vi "HFCalibrate.vi"(7 "error in (no error)":errorcluster, 10 "VISA resource name":refnum<visa-resource-name>) -> (0 "error out":errorcluster, 1 "Calibrated freq / Hz":dbl, 2 "Calibration factor":dbl, 3 "VISA resource name out":refnum<visa-resource-name>)   [LabVIEW 2017, in "GP22_TDC_Arduinoed.lvlib"]
doc: "Calibrate the high frequency clokc by comparing it to the low freq but very stable 32.768 kHz clock.\n\nThis stores and returns a correction factor for the HF clock: e.g. if the clock is nominally 4MHz with a correction factor of 1.005, the true freq. is 4.02MHz. \n\nThe return value can be safely ignored: it is automatically stored and used by the measurement subVIs to calibrate their readings.\n\nCompared to the TDC calibration, this takes much longer and should be performed less often. TDC calibration should be carried out every few hundred measurements, but HF resonator calibration needs only to be done at the start of a measurement run. \n\nNote that this calibration is not handled automatically by the GP22 chip evenin \"autocalibrate\" mode, and so is dealt with by Labview."
uses:
  GP22_TDC_Arduinoed.lvlib
  Globals.vi
panel:
  out "read buffer":string
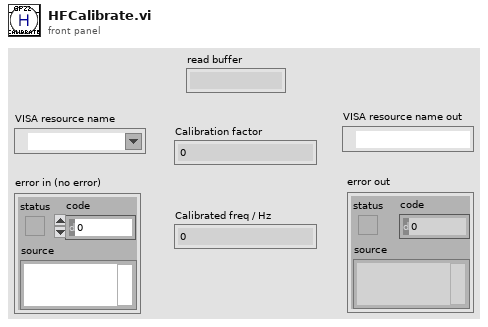
[diagram p1: front panel]
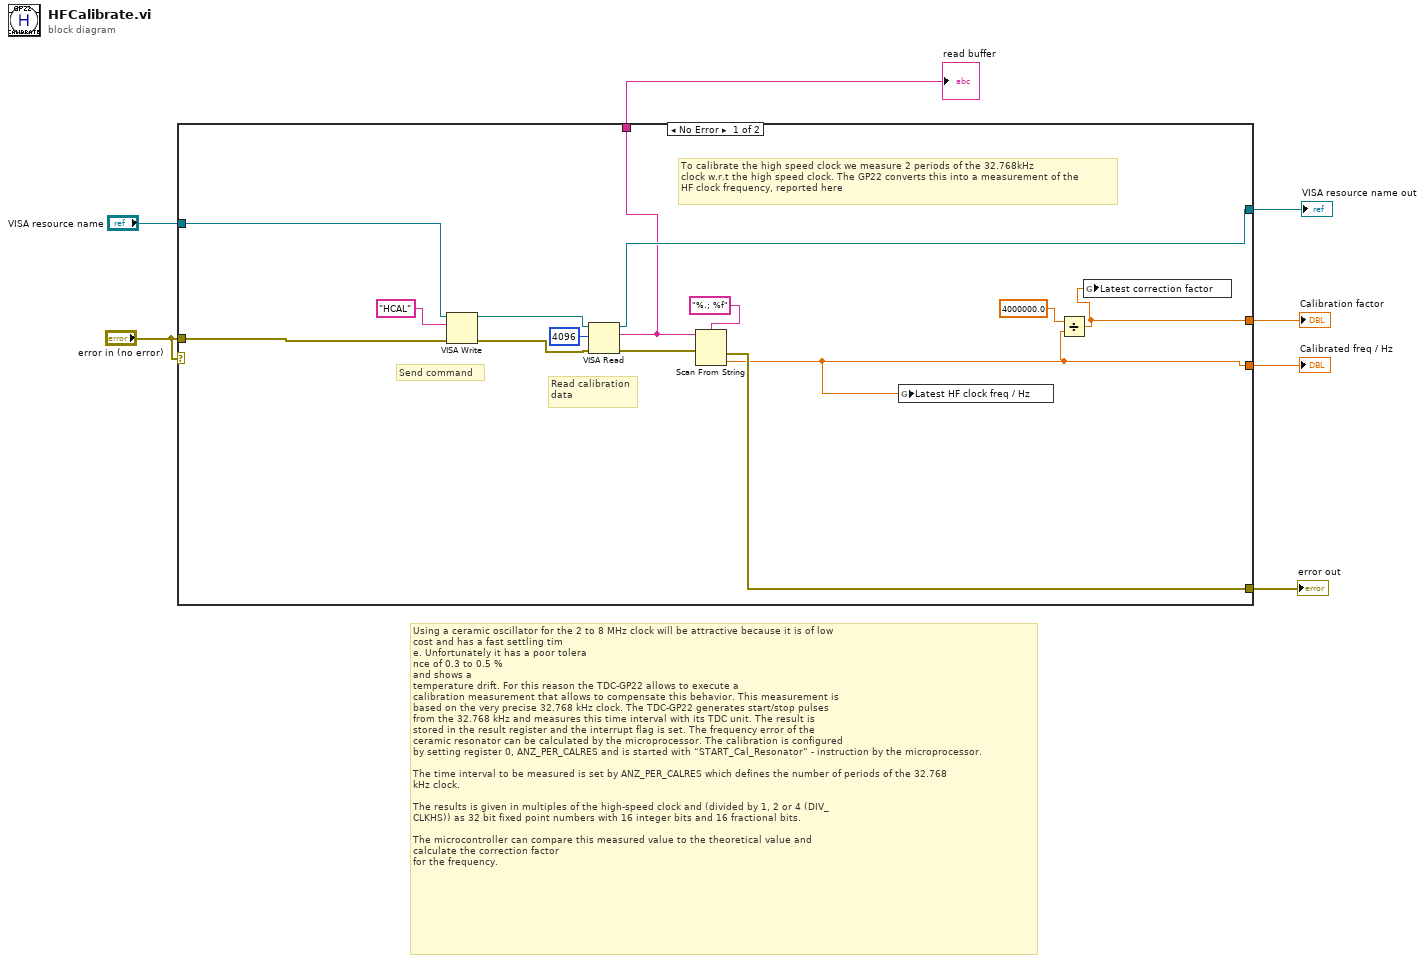
[diagram p0: block diagram]
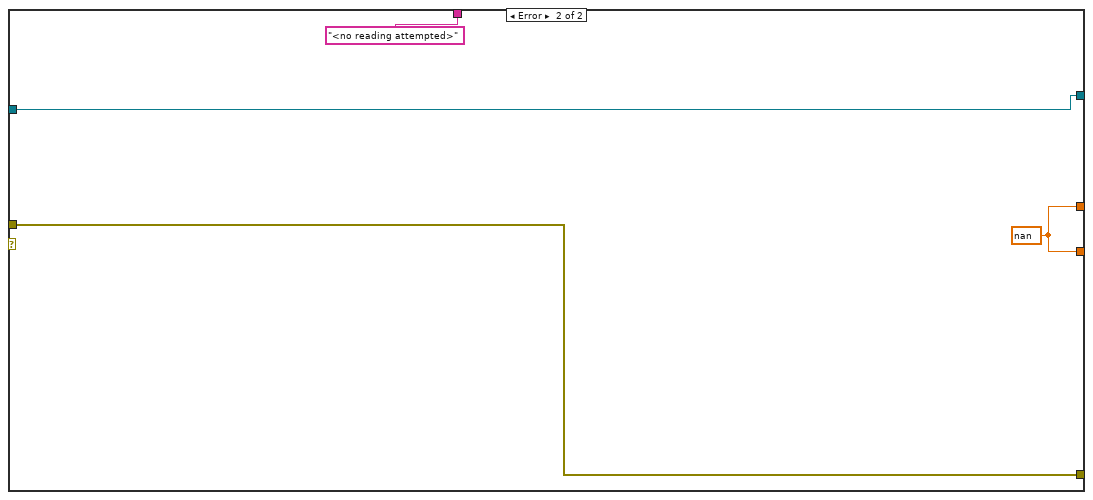
[diagram p2: hidden frame]
diagram:
  # "Using a ceramic oscillator for the 2 to 8 MHz clock will be attractive because it is of low\ncost and has a fast settling tim\ne. Unfortunately it has a poor tolera\nnce of 0.3 to 0.5 %\nand shows a\ntemperature drift. For this reason the TDC-GP22 allows to execute a\ncalibration measurement that allows to compensate this behavior. This measurement is\nbased on the very precise 32.768 kHz clock. The TDC-GP22 generates start/stop pulses\nfrom the 32.768 kHz and measures this time interval with its TDC unit. The result is\nstored in the result register and the interrupt flag is set. The frequency error of the\nceramic resonator can be calculated by the microprocessor. The calibration is configured\nby setting register 0, ANZ_PER_CALRES and is started with “START_Cal_Resonator“ - instruction by the microprocessor.\n\nThe time interval to be measured is set by ANZ_PER_CALRES which defines the number of periods of the 32.768\nkHz clock.\n\nThe results is given in multiples of the high-speed clock and (divided by 1, 2 or 4 (DIV_\nCLKHS)) as 32 bit fixed point numbers with 16 integer bits and 16 fractional bits.\n\nThe microcontroller can compare this measured value to the theoretical value and\ncalculate the correction factor\nfor the frequency."
  n1 = case shown="No Error" "error in (no error)" {
    tunnel: "error in (no error)" -> [w21 w25]
    tunnel: [w15 w25] -> w7
    tunnel: "VISA resource name" -> [w13 w23]
    tunnel: [w12 w23] -> w4
    tunnel: [w11 "<no reading attempted>" ("read buffer")] -> w3
    tunnel: [w8 w24] -> w2
    tunnel: [w9 w24] -> w1
    frame No Error {
      # "To calibrate the high speed clock we measure 2 periods of the 32.768kHz\nclock w.r.t the high speed clock. The GP22 converts this into a measurement of the\nHF clock frequency, reported here"
      # "Read calibration\ndata"
      # "Send command"
      n2 = VISA Write(VISA resource name=w13, write buffer="HCAL" ("command"), error in (no error)=w21) -> (VISA resource name out=w14:refnum<visa-resource-name>, error out=w20:errorcluster)  [unwired: 1 out]
      n3 = VISA Read(VISA resource name=w14, byte count=u32 4096, error in (no error)=w20) -> (VISA resource name out=w12:refnum<visa-resource-name>, read buffer=w11:string, error out=w16:errorcluster)  [unwired: 1 out]
      n4 = Scan From String(format string="%.; %f", input string=w11, error in=w16) -> (error out=w15:errorcluster, output 1=w9:dbl)  [unwired: 2 in, 2 out]
      n5 = global write "Globals.vi" "Latest HF clock freq / Hz"(w9) -> ()
      n6 = Divide(x=4000000.0, y=w9) -> (x/y=w8:dbl)
      n7 = global write "Globals.vi" "Latest correction factor"(w8) -> ()
    }
    frame Error {
      w24 = nan
    }
  }
  "error out" <- w7
  "VISA resource name out" <- w4
  "read buffer" <- w3
  "Calibration factor" <- w2
  "Calibrated freq / Hz" <- w1
